vi "dsmm-registrationLowLevel.vi"(0 "X":dbl[][](array[numeric]), 1 "allocate":bool=TRUE, 2 "allocate_size":i32=90000, 5 "Y":dbl[][](array[numeric]), 7 "beta":dbl=2.0, 9 "lambda":dbl=1.5, 11 "neighbor_cutoff":dbl=10.0, 12 "alpha":dbl=1.0, 13 "conv_epsilon":dbl=0.001) -> (4 "X out":dbl[][](array[numeric]), 6 "Y out":dbl[][](array[numeric]), 10 "p":dbl[][](array[numeric]))   [LabVIEW 2017]
uses:
  dll/wormUtilities/x64/Release/wormUtilities.dll
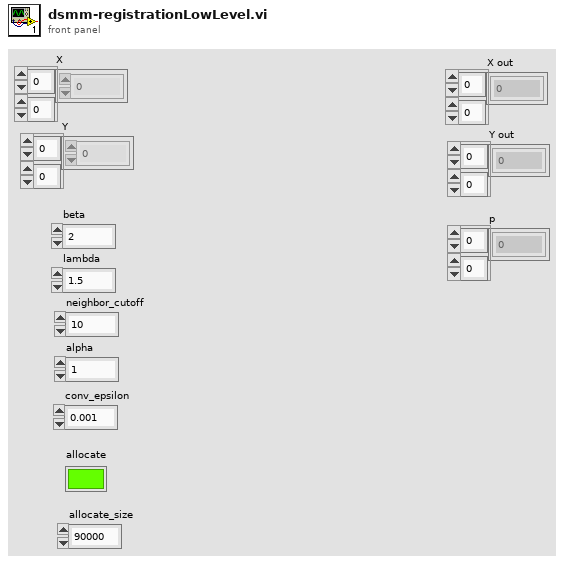
[diagram p1: front panel]
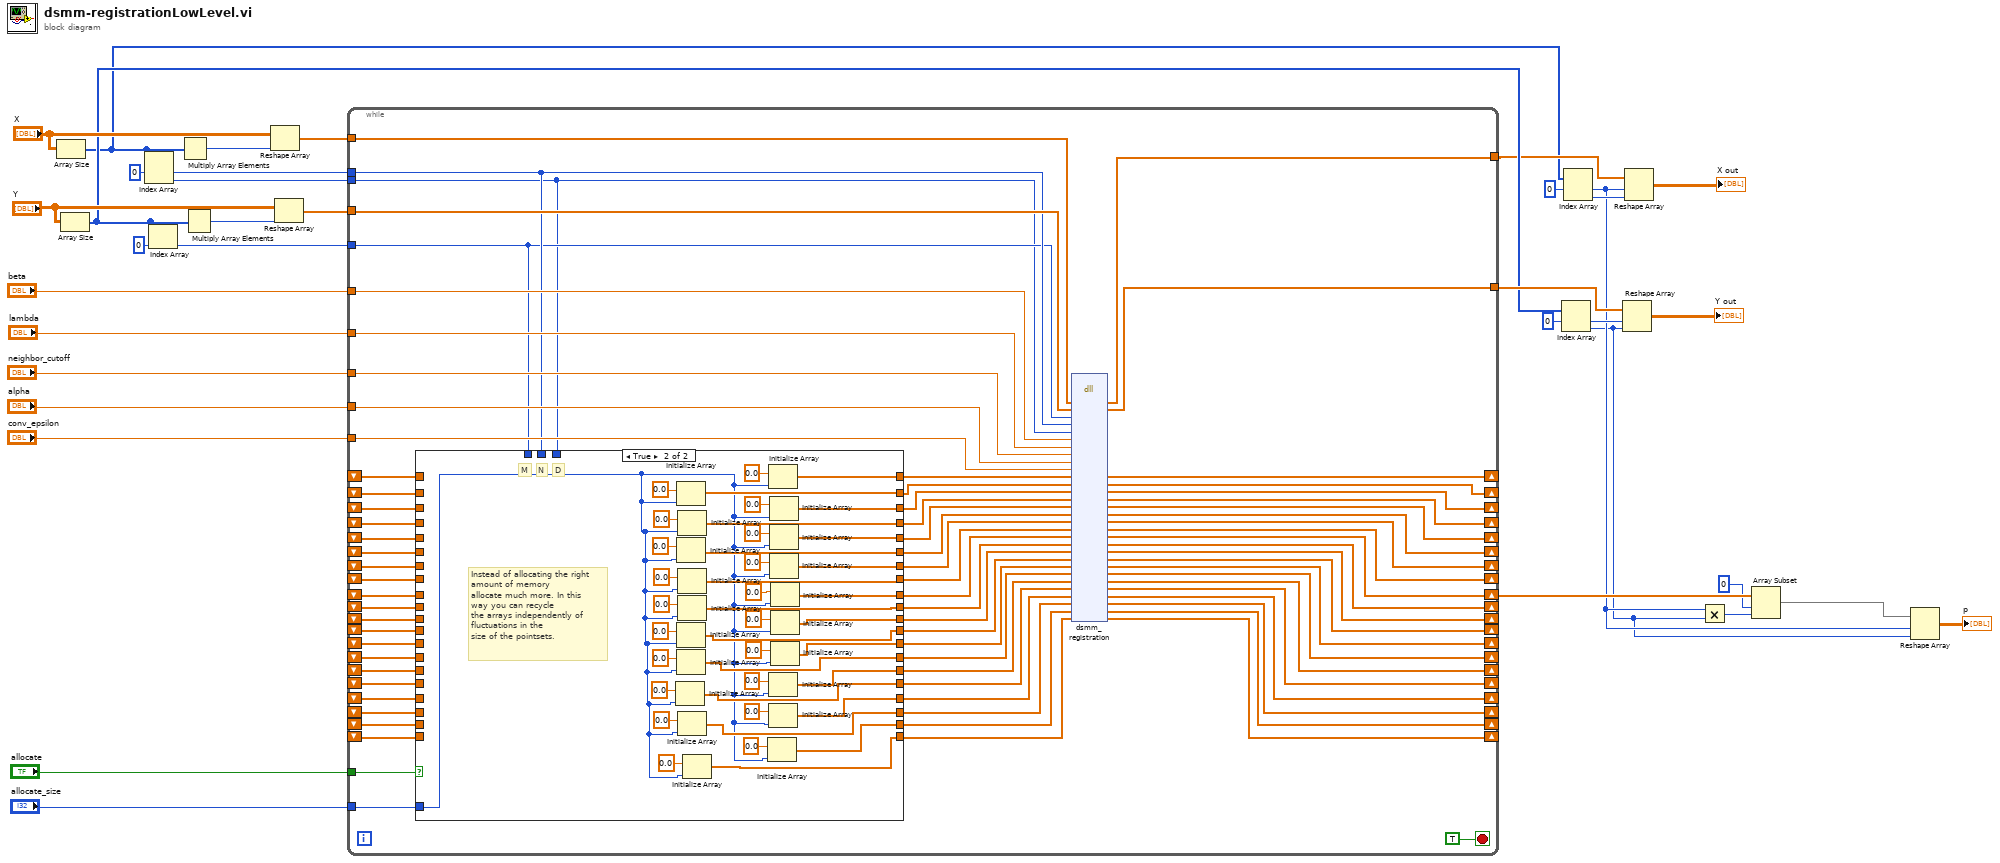
[diagram p0: block diagram]
diagram:
  n1 = Array Size(array="X") -> (size(s)=w4:i32[])
  n2 = Array Size(array="Y") -> (size(s)=w10:i32[])
  n3 = Index Array(array=w4, index #1=0 ("index")) -> (element #1=w26:i32, element #2=w25:i32)  [unwired: 1 in]
  n4 = Index Array(array=w10, index=0) -> (element=w20:i32)
  n5 = Multiply Array Elements(1:w4) -> (0:w28:i32)
  n6 = Multiply Array Elements(1:w10) -> (0:w24:i32)
  n7 = Reshape Array("X", w28) -> (w27:dbl[])
  n8 = Reshape Array("Y", w24) -> (w21:dbl[])
  n9 = while {
    tunnel: "beta" -> [w110]
    tunnel: "lambda" -> [w109]
    tunnel: "neighbor_cutoff" -> [w108]
    tunnel: "alpha" -> [w107]
    tunnel: "conv_epsilon" -> [w106]
    tunnel: [w105] -> w15
    tunnel: w27 -> [w103]
    tunnel: w26 -> [w41]
    tunnel: w25 -> [w39]
    tunnel: w21 -> [w102]
    tunnel: w20 -> [w40]
    shift-right: [w101] -> _
    shift-left: _ -> [w82]
    shift-right: [w100] -> _
    shift-left: _ -> [w80]
    shift-right: [w99] -> _
    shift-left: _ -> [w78]
    shift-right: [w98] -> _
    shift-left: _ -> [w77]
    shift-right: [w97] -> _
    shift-left: _ -> [w75]
    shift-right: [w96] -> _
    shift-left: _ -> [w74]
    shift-right: [w95] -> _
    shift-left: _ -> [w70]
    shift-right: [w94] -> _
    shift-left: _ -> [w68]
    shift-right: [w104] -> w13
    shift-left: _ -> [w66]
    shift-right: [w93] -> _
    shift-left: _ -> [w64]
    shift-right: [w92] -> _
    shift-left: _ -> [w62]
    shift-right: [w91] -> _
    shift-left: _ -> [w60]
    shift-right: [w90] -> _
    shift-left: _ -> [w58]
    shift-right: [w89] -> _
    shift-left: _ -> [w56]
    shift-right: [w88] -> _
    shift-left: _ -> [w54]
    shift-right: [w87] -> _
    shift-left: _ -> [w52]
    shift-right: [w86] -> _
    shift-left: _ -> [w50]
    shift-right: [w85] -> _
    shift-left: _ -> [w48]
    shift-right: [w84] -> _
    shift-left: _ -> [w46]
    shift-right: [w83] -> _
    shift-left: _ -> [w44]
    tunnel: "allocate" -> [w42]
    tunnel: "allocate_size" -> [w38]
    tunnel: [w36] -> w5
    stop <- TRUE stop-if-true
    n10 = case shown="True" w42 {
      tunnel: w82 -> [w130 _]
      tunnel: [w130 w170] -> w81
      tunnel: w80 -> [w129 _]
      tunnel: [w129 w168] -> w79
      tunnel: w78 -> [w111 _]
      tunnel: [w111 w166] -> w71
      tunnel: w77 -> [w128 _]
      tunnel: [w128 w164] -> w76
      tunnel: w75 -> [w112 _]
      tunnel: [w112 w162] -> w72
      tunnel: w74 -> [w127 _]
      tunnel: [w127 w156] -> w73
      tunnel: w70 -> [w126 _]
      tunnel: [w126 w160] -> w69
      tunnel: [w125 w154] -> w67
      tunnel: w68 -> [w125 _]
      tunnel: [w124 w158] -> w65
      tunnel: w66 -> [w124 _]
      tunnel: [w123 w152] -> w63
      tunnel: w64 -> [w123 _]
      tunnel: [w122 w150] -> w61
      tunnel: w62 -> [w122 _]
      tunnel: w60 -> [w121 _]
      tunnel: [w121 w148] -> w59
      tunnel: w58 -> [w120 _]
      tunnel: [w120 w146] -> w57
      tunnel: w56 -> [w119 _]
      tunnel: [w119 w144] -> w55
      tunnel: w54 -> [w118 _]
      tunnel: [w118 w142] -> w53
      tunnel: w52 -> [w117 _]
      tunnel: [w117 w140] -> w51
      tunnel: w50 -> [w116 _]
      tunnel: [w116 w138] -> w49
      tunnel: w48 -> [w115 _]
      tunnel: [w115 w136] -> w47
      tunnel: w46 -> [w114 _]
      tunnel: [w114 w134] -> w45
      tunnel: w44 -> [w113 _]
      tunnel: [w113 w132] -> w43
      tunnel: w41 -> [_ _]
      tunnel: w40 -> [_ _]
      tunnel: w39 -> [_ _]
      tunnel: w38 -> [_ w131]
      frame False {
      }
      frame True {
        # "Instead of allocating the right amount of memory\nallocate much more. In this way you can recycle\nthe arrays independently of fluctuations in the \nsize of the pointsets."
        # "D"
        # "N"
        # "M"
        n11 = Initialize Array(0.0 ("element"), w131) -> (w140:dbl[])
        n12 = Initialize Array(0.0 ("element"), w131) -> (w168:dbl[])
        n13 = Initialize Array(0.0 ("element"), w131) -> (w156:dbl[])
        n14 = Initialize Array(0.0 ("element"), w131) -> (w148:dbl[])
        n15 = Initialize Array(0.0 ("element"), w131) -> (w144:dbl[])
        n16 = Initialize Array(0.0 ("element"), w131) -> (w164:dbl[])
        n17 = Initialize Array(0.0 ("element"), w131) -> (w154:dbl[])
        n18 = Initialize Array(0.0 ("element"), w131) -> (w152:dbl[])
        n19 = Initialize Array(0.0 ("element"), w131) -> (w136:dbl[])
        n20 = Initialize Array(0.0 ("element"), w131) -> (w132:dbl[])
        n21 = Initialize Array(0.0 ("element"), w131) -> (w134:dbl[])
        n22 = Initialize Array(0.0 ("element"), w131) -> (w170:dbl[])
        n23 = Initialize Array(0.0 ("element"), w131) -> (w142:dbl[])
        n24 = Initialize Array(0.0 ("element"), w131) -> (w138:dbl[])
        n25 = Initialize Array(0.0 ("element"), w131) -> (w166:dbl[])
        n26 = Initialize Array(0.0 ("element"), w131) -> (w162:dbl[])
        n27 = Initialize Array(0.0 ("element"), w131) -> (w160:dbl[])
        n28 = Initialize Array(0.0 ("element"), w131) -> (w158:dbl[])
        n29 = Initialize Array(0.0 ("element"), w131) -> (w150:dbl[])
        n30 = Initialize Array(0.0 ("element"), w131) -> (w146:dbl[])
      }
    }
    n31 = dll-call lib="C:/Users/francesco/dev/pump-probe/dll/wormUtilities/x64/Release/wormUtilities.dll" fn="dsmm_registration"("X"=w103, "Y"=w102, "M"=w40, "N"=w41, "D"=w39, "beta"=w110, "lambda"=w109, "neighbor_cutoff"=w108, "alpha"=w107, "conv_epsilon"=w106, "pwise_dist"=w81, "pwise_distYY"=w79, "Gamma"=w71, "CDE_term"=w76, "w"=w72, "F_t"=w73, "wF_t"=w69, "wF_t_sum"=w67, "p"=w65, "u"=w63, "hatP"=w61, "hatPI_diag"=w59, "hatPIG"=w57, "hatPX"=w55, "hatPIY"=w53, "G"=w51, "W"=w49, "GW"=w47, "sumPoverN"=w45, "expAlphaSumPoverN"=w43) -> ("X"=w36:dbl[], "Y"=w105:dbl[], "pwise_dist"=w101:dbl[], "pwise_distYY"=w100:dbl[], "Gamma"=w99:dbl[], "CDE_term"=w98:dbl[], "w"=w97:dbl[], "F_t"=w96:dbl[], "wF_t"=w95:dbl[], "wF_t_sum"=w94:dbl[], "p"=w104:dbl[], "u"=w93:dbl[], "hatP"=w92:dbl[], "hatPI_diag"=w91:dbl[], "hatPIG"=w90:dbl[], "hatPX"=w89:dbl[], "hatPIY"=w88:dbl[], "G"=w87:dbl[], "W"=w86:dbl[], "GW"=w85:dbl[], "sumPoverN"=w84:dbl[], "expAlphaSumPoverN"=w83:dbl[])  [unwired: 12 in, 2 out]
  }
  n32 = Index Array(array=w10, index #1=0 ("index")) -> (element #1=w16:i32, element #2=w1:i32)  [unwired: 1 in]
  n33 = Index Array(array=w4, index #1=0 ("index")) -> (element #1=w2:i32, element #2=w7:i32)  [unwired: 1 in]
  n34 = Reshape Array(w15, w16, w1) -> (→"Y out":dbl[][])
  n35 = Reshape Array(w5, w2, w7) -> (→"X out":dbl[][])
  n36 = Multiply(x=w2, y=w1) -> (x*y=w3:i32)
  n37 = Array Subset(array=w13, index=0, length=w3) -> (w11:dbl[])
  n38 = Reshape Array(w11, w2, w1) -> (→"p":dbl[][])
